vi "Query Input Attenuation Resolution.vi"(8 "error in (no error)":errorcluster, 10 "Platform Slot Number (10)":i16=10 min=-1 max=255, 11 "VISA resource name":refnum<visa-resource-name>) -> (0 "error out":errorcluster, 2 "Attenuation Resolution":dbl format="%#_6e", 3 "VISA resource name out":refnum<visa-resource-name>)   [LabVIEW 2018, in "LTB-1.lvlib" / "3150.lvlib"]
doc: "Queries the smallest attenuation step available. It determines the maximum resolution of the attenuation."
uses:
  3150.lvlib
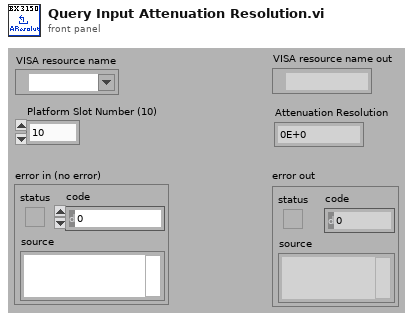
[diagram p1: front panel]
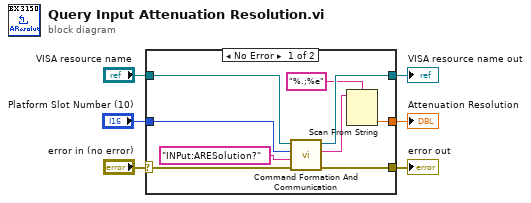
[diagram p0: block diagram]
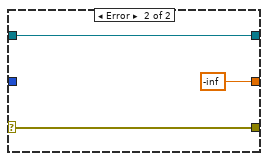
[diagram p2: hidden frame]
diagram:
  n1 = case shown="No Error" "error in (no error)" {
    selector: "error in (no error)" -> [w15 w18]
    tunnel: [w14 w18] -> w4
    tunnel: "VISA resource name" -> [w12 w17]
    tunnel: [w11 w17] -> w5
    tunnel: "Platform Slot Number (10)" -> [w10 _]
    tunnel: [w8 -inf] -> w1
    frame No Error {
      n2 = call "Command Formation And Communication.vi"("error in (no error)"=w15, "Command"="INPut:ARESolution?", "Platform Slot Number"=w10, "VISA resource name"=w12) -> ("error out"=w14:errorcluster, "Response"=w9:string, "VISA resource name out"=w11:refnum<visa-resource-name>)  [unwired: 5 out]
      n3 = Scan From String(format string="%.;%e", input string=w9) -> (output 1=w8:dbl)  [unwired: 2 in, 4 out]
    }
    frame Error {
    }
  }
  "VISA resource name out" <- w5
  "error out" <- w4
  "Attenuation Resolution" <- w1
